vi "elevatorStuffs.vi"   [LabVIEW 2014]
uses:
  Support Files/ElevatorStates.ctl
  Support Files/DropStates.ctl
  Support Files/RC PickupStates.ctl
  Support Files/TransitionStates.ctl
  Support Files/HandOffStates.ctl
  Support Files/FeederModeStates.ctl
  Support Files/FeederModePickUpStates.ctl
  Support Files/FeederModeStartStates.ctl
  Support Files/Global Data!!!.vi
types:
  T1 = typedef "ElevatorStates.ctl" = enum16{"DropSequence", "Reset", "Drop1Stage", "2StageEngage", "Lift1Stage", "1StageEngage", "Rest", "InterruptedLift", "Manual", "Auto2Man", "Initialize", "FeederMode"}
  T2 = typedef "DropStates.ctl" = enum16{"Lower", "Retract", "Release", "Drop1Inch", "Not", "Reset", "Pause", "isArmOut", "putArmOut"}
  T3 = typedef "RC PickupStates.ctl" = enum16{"PickToteUp", "Disengage", "Drop", "Hold", "Lift", "Engage1Stage", "Rest", "DropAgain", "Done", "Lift.5", "Pause4Jones"}
  T4 = typedef "TransitionStates.ctl" = enum16{"Release 2 Stage", "Hand-Off", "Do Nothing"}
  T5 = typedef "HandOffStates.ctl" = enum16{"Done", "Release2Stage", "Engage1Stage", "Raise1Stage", "Pause"}
  T6 = typedef "FeederModePickUpStates.ctl" = enum16{"ToEnding", "Pick Up", "Engage", "DropDown", "Release", "Drop", "Wait", "Engage2Stage", "Disengage2Stage"}
  T7 = typedef "FeederModeStates.ctl" = enum16{"Ending", "PickUp", "Starting", "Reset"}
  T8 = typedef "FeederModeStartStates.ctl" = enum16{"ToPickUp", "LiftUp", "Engage", "Wait", "Lift", "Release", "Drop"}
  T9 = typedef "WPI_SwitchDevRef.ctl" = cluster{"DevStatus":errorcluster, "DIO Channel":T10, "Controller":T11, "CntIndex":T12, "Normally Closed":bool}
  T10 = typedef "FPGA_DIOChannel.ctl" = enum8{"DIO 0", "DIO 1", "DIO 2", "DIO 3", "DIO 4", "DIO 5", "DIO 6", "DIO 7", "DIO 8", "DIO 9", "DIO MXP 0", "DIO MXP 1", "DIO MXP 2", "DIO MXP 3", "DIO MXP 4", "DIO MXP 5", "DIO MXP 6", "DIO MXP 7", "DIO MXP 8", "DIO MXP 9", "DIO MXP 10", "DIO MXP 11", "DIO MXP 12", "DIO MXP 13", "DIO MXP 14", "DIO MXP 15", "Invalid"}
  T11 = typedef "FPGA_TypedefDigitalModule.ctl" = enum16{"Controller 1"}
  T12 = typedef "FPGA_CounterCtrSystemIndex.ctl" = enum8{"Ctr 0", "Ctr 1", "Ctr 2", "Ctr 3", "Ctr 4", "Ctr 5", "Ctr 6", "Ctr 7", "Invalid"}
  T13 = typedef "WPI_EncoderDevRef.ctl" = cluster{"DevStatus":errorcluster, "EncoderIndex":T14, "CounterIndex":T12, "DistancePerCount":dbl, "Decoding Type":T15}
  T14 = typedef "FPGA_EncoderIdx.ctl" = enum8{"Enc 0", "Enc 1", "Enc 2", "Enc 3", "Enc 4", "Enc 5", "Enc 6", "Enc 7", "Invalid"}
  T15 = typedef "WPI_EncoderType.ctl" = enum16{"1x", "2x", "4x"}
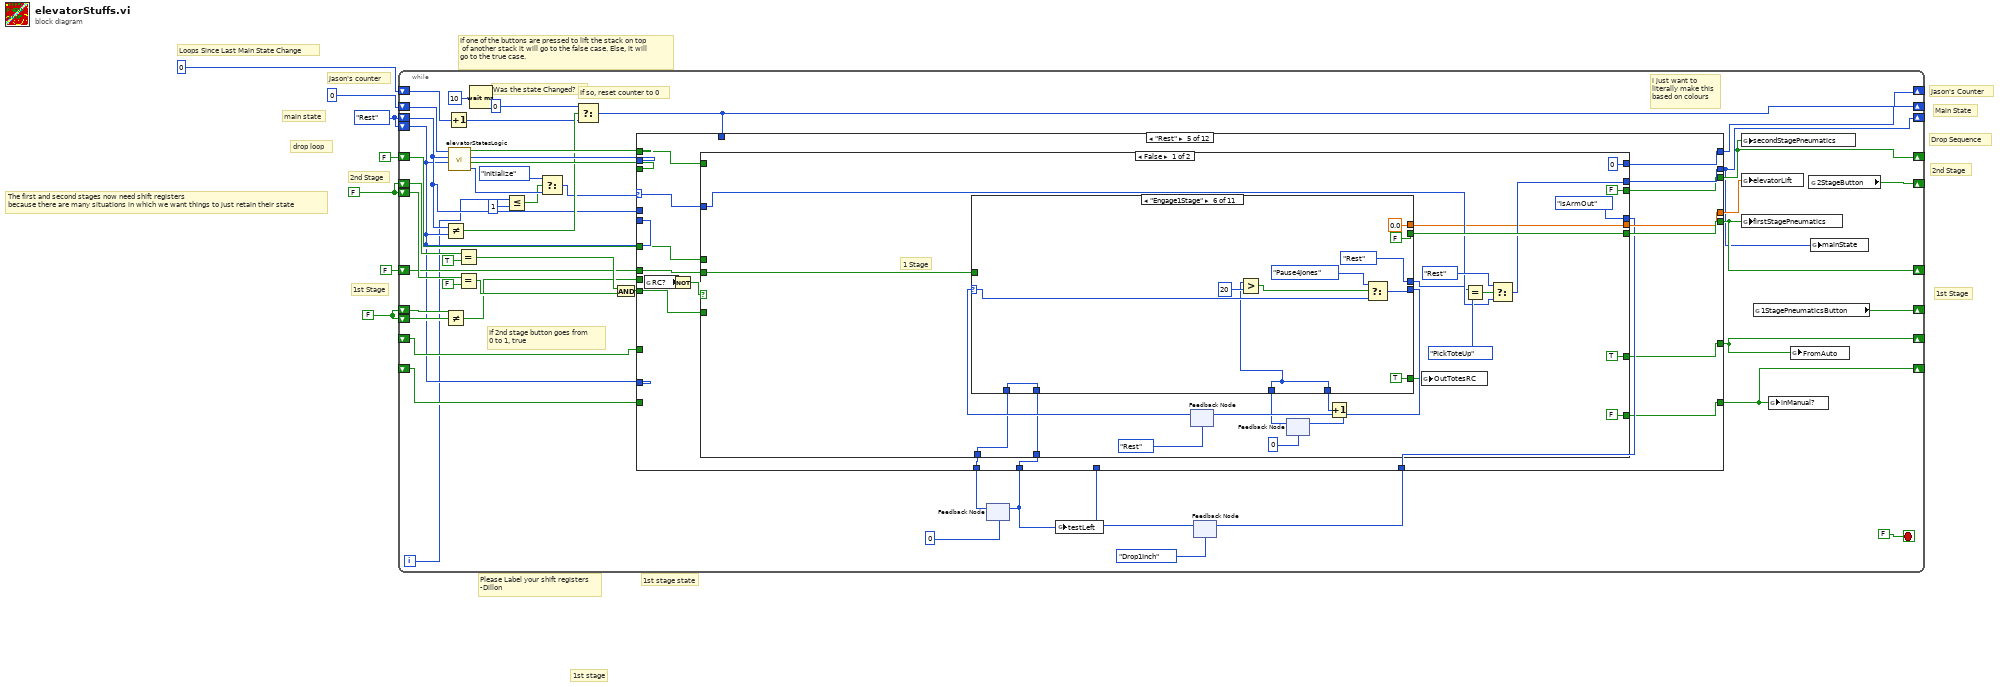
[diagram p0: block diagram]
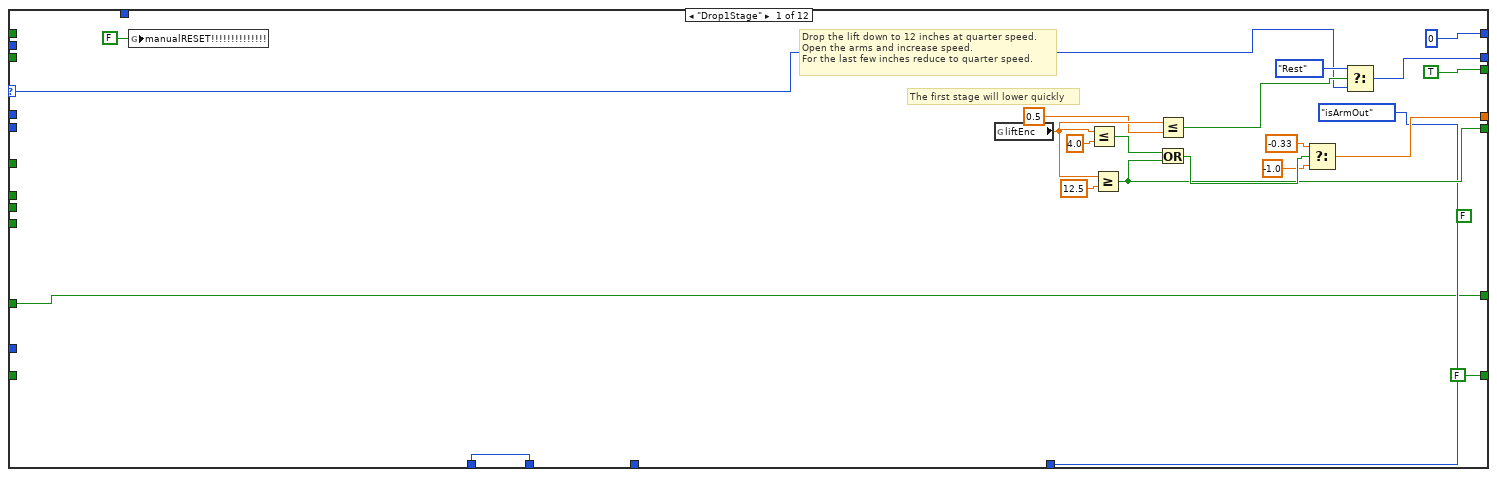
[diagram p2: hidden frame]
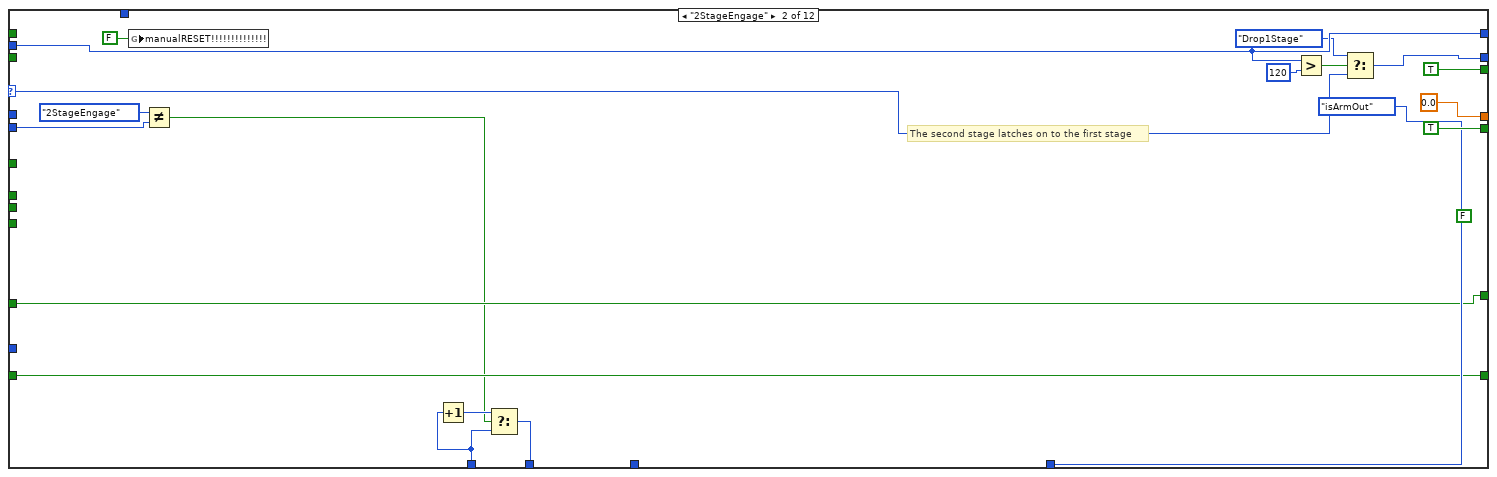
[diagram p3: hidden frame]
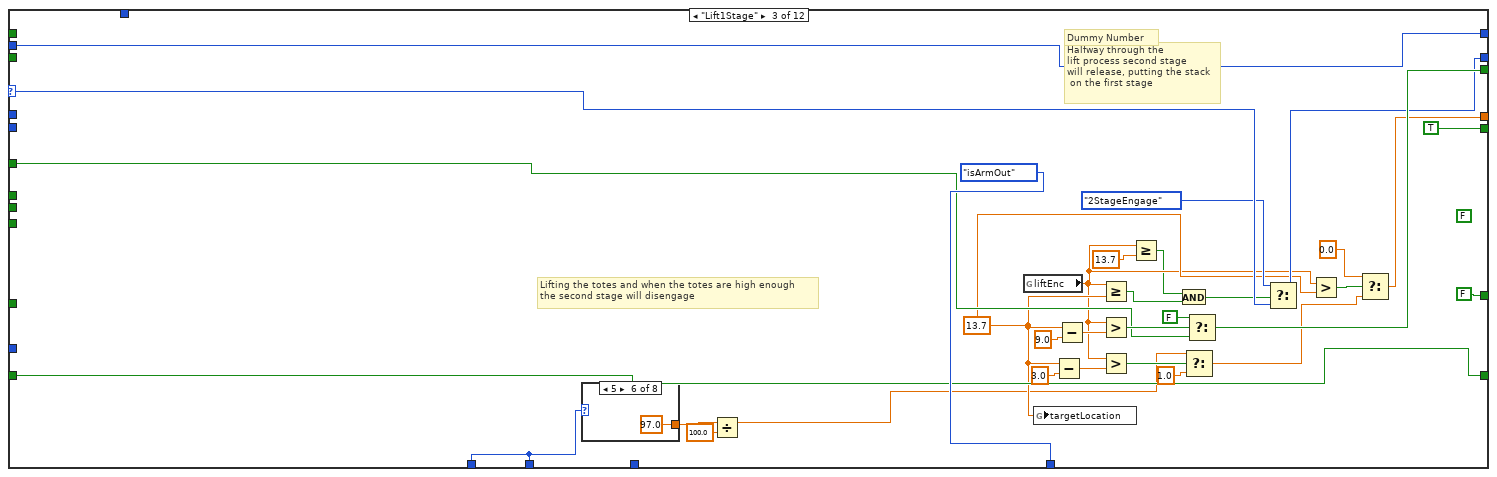
[diagram p4: hidden frame]
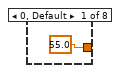
[diagram p5: hidden frame]
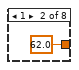
[diagram p6: hidden frame]
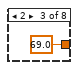
[diagram p7: hidden frame]
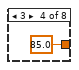
[diagram p8: hidden frame]
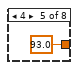
[diagram p9: hidden frame]
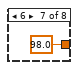
[diagram p10: hidden frame]
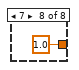
[diagram p11: hidden frame]
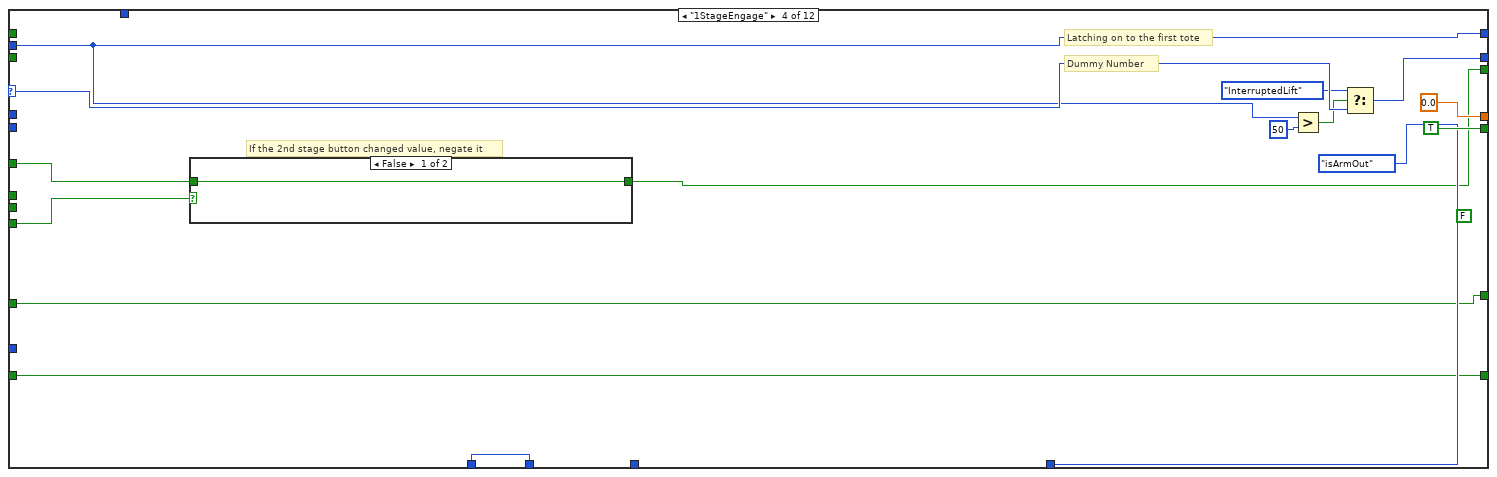
[diagram p12: hidden frame]
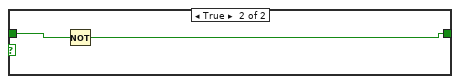
[diagram p13: hidden frame]
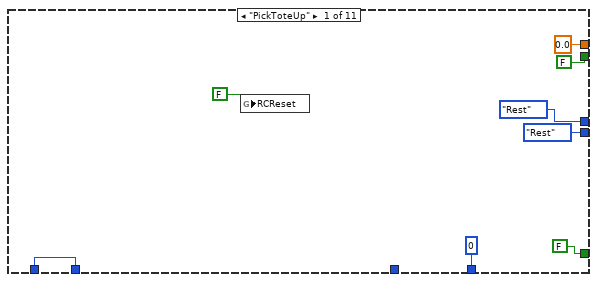
[diagram p14: hidden frame]
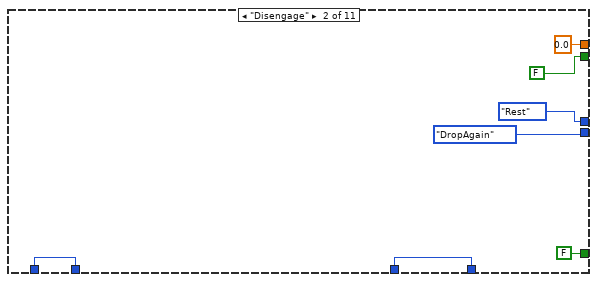
[diagram p15: hidden frame]
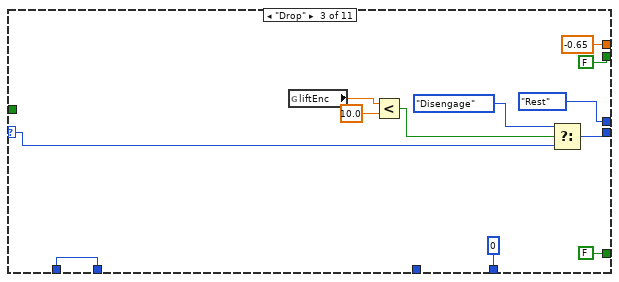
[diagram p16: hidden frame]
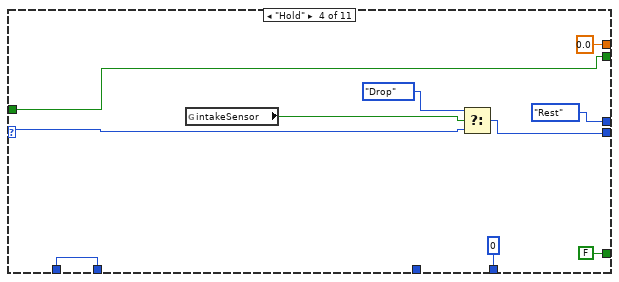
[diagram p17: hidden frame]
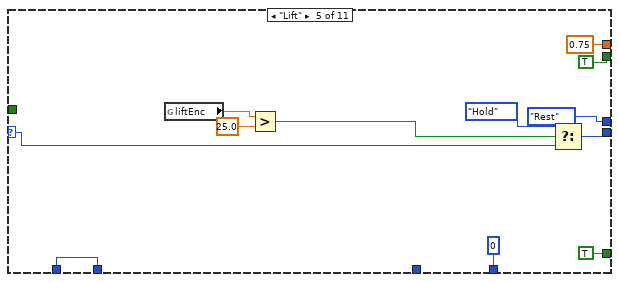
[diagram p18: hidden frame]
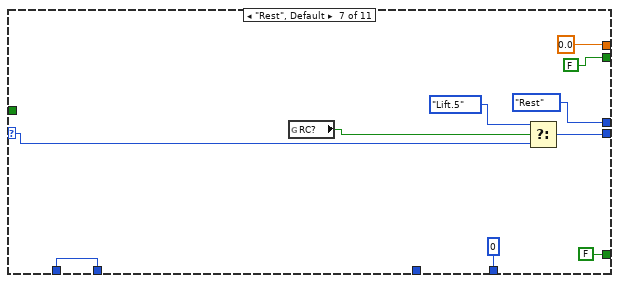
[diagram p19: hidden frame]
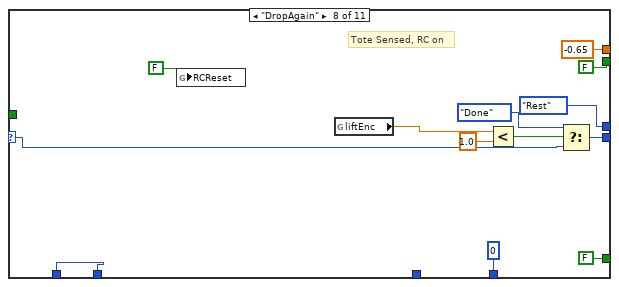
[diagram p20: hidden frame]
diagram:
  w1 = FALSE ("1StagePneumaticsButton")
  w3 = FALSE ("2StageButton")
  w6 = ElevatorStates."Rest" ("Enum")
  # "Jason's Counter"
  # "Main State"
  # "Drop Sequence"
  # "The first and second stages now need shift registers\nbecause there are many situations in which we want things to just retain their state"
  # "main state"
  # "drop loop"
  # "2nd Stage"
  # "1st Stage"
  # "1st Stage"
  # "1st stage state"
  # "1st stage"
  # "2nd Stage"
  # "Jason's counter"
  # "Loops Since Last Main State Change"
  # "Please Label your shift registers\n-Dillon"
  # "If one of the buttons are pressed to lift the stack on top\n of another stack it will go to the false case. Else, it will\ngo to the true case."
  n1 = while {
    shift-right: [w23] -> _
    shift-left: w6 -> [w15]
    shift-right: [w53] -> _
    shift-left: 0 -> [w55]
    shift-left: w6 -> [w14]
    shift-right: [w27] -> _
    shift-left: 0 -> [w44]
    shift-right: [w43] -> _
    shift-left: FALSE ("t") -> [w42]
    shift-right: [w41] -> _
    shift-left: w3 -> [w40]
    shift-left: w3 -> [w36]
    shift-right: [w33] -> _
    shift-left: FALSE ("f") -> [w28]
    shift-right: [w32] -> _
    shift-left: w1 -> [w31]
    shift-left: w1 -> [w30]
    shift-right: [w22] -> _
    shift-left: _ -> [w21]
    shift-right: [w20] -> _
    shift-left: _ -> [w19]
    i -> [w9]
    stop <- FALSE stop-if-true
    # "If 2nd stage button goes from\n0 to 1, true"
    # "If so, reset counter to 0"
    # "Was the state Changed?"
    # "i just want to \nliterally make this\nbased on colours"
    n2 = Not Equal?(x=w15, y=w14) -> (x != y?=w47:bool)
    n3 = Not Equal?(x=w31, y=w30) -> (x != y?=w29:bool)
    n4 = Increment(x=w44) -> (x+1=w45:i32)
    n5 = call "elevatorStatesLogic.vi"("oldState"=w14, "newState"=w15, "timer"=w55) -> ("State"=w12:T1, "manual?"=w48:bool, "Numeric"=w54:i32, "elevatorActive"=w49:bool)  [unwired: 5 in]
    n6 = Equal?(x=w40, y=TRUE) -> (x = y?=w38:bool)
    n7 = Equal?(x=w36, y=FALSE) -> (x = y?=w37:bool)
    n8 = Wait (ms)(milliseconds to wait=u32 10) -> ()  [unwired: 1 out]
    n9 = Less Or Equal?(x=w9, y=1) -> (x <= y?=w10:bool)
    n10 = Select(t=ElevatorStates."Initialize", s=w10, f=w12) -> (s? t:f=w13:T1)
    n11 = Select(t=0, s=w47, f=w45) -> (s? t:f=w27:i32)
    n12 = And(x=w38, y=w37) -> (x .and. y?=w39:bool)
    n13 = feedback #1(0) -> (w17:i32)
    n14 = feedback #2(DropStates."Drop1Inch" ("Enum")) -> (w25:T2)
    n15 = case shown="\"Rest\"" w13 {
      selector: w13 -> [w72 w92 w122 w148 w161 w337 w357 w399 w440 w561 _ w673]
      tunnel: [w71 w89 w120 w143 w167 w336 w367 w411 w432 w562 ElevatorStates."Rest" ("Enum") w672] -> w23
      tunnel: [w70 0.0 w108 0.0 w169 w335 w365 w386 w442 w552 0.0 ("f") w670] -> w52
      tunnel: [w62 TRUE TRUE TRUE w170 w332 TRUE ("t") w376 w439 w551 FALSE ("Stage1?") w669] -> w33
      tunnel: [TRUE TRUE ("t") w125 w139 w164 FALSE ("t") w345 FALSE ("t") FALSE ("t") w548 FALSE ("t") w652] -> w43
      tunnel: w54 -> [_ w91 w123 w145 _ _ _ _ w436 w550 _ _]
      tunnel: [0 ("t") w91 w123 w145 w168 0 ("t") 0 ("t") 0 ("t") w437 w546 0 ("Numeric") 0 ("Numeric")] -> w53
      tunnel: w49 -> [_ _ _ _ w166 _ _ _ _ _ _ _]
      tunnel: w25 -> [_ _ _ _ _ _ _ _ w441 w558 _ _]
      tunnel: [DropStates."isArmOut" ("Enum") DropStates."isArmOut" ("Enum") DropStates."isArmOut" ("Enum") DropStates."isArmOut" ("Enum") w165 DropStates."isArmOut" ("Enum") DropStates."isArmOut" ("Enum") DropStates."isArmOut" ("Enum") w438 w558 DropStates."isArmOut" ("Enum") DropStates."isArmOut" ("Enum")] -> w24
      tunnel: w48 -> [_ _ _ _ _ _ _ w385 _ _ _ _]
      tunnel: w14 -> [_ _ _ _ _ _ _ w383 _ _ _ _]
      tunnel: w42 -> [_ _ w112 w141 w163 _ w345 w379 _ _ _ _]
      tunnel: w39 -> [_ _ _ w140 w162 _ _ w380 w430 _ _ _]
      tunnel: w29 -> [_ _ _ _ _ _ _ w378 _ _ _ _]
      tunnel: w28 -> [_ _ _ _ w158 w332 _ w377 _ _ _ _]
      tunnel: w27 -> [_ _ _ _ _ _ _ _ w429 _ _ _]
      tunnel: [FALSE w84 w111 w138 w160 FALSE w348 TRUE w428 w559 FALSE FALSE] -> w22
      tunnel: w21 -> [_ w84 w111 w138 _ _ w348 _ w428 w559 _ _]
      tunnel: [w57 w83 FALSE w137 w159 FALSE TRUE w374 FALSE w539 TRUE FALSE] -> w20
      tunnel: w19 -> [w57 w83 _ w137 _ _ _ w374 _ _ _ _]
      tunnel: w17 -> [w56 w81 w99 w136 w155 w329 w346 w373 _ w547 w644 w682]
      tunnel: [w56 w79 w99 w136 w154 w329 w346 w373 0 w547 w644 w682] -> w16
      tunnel: w15 -> [_ _ _ _ _ _ _ _ _ _ _ _]
      tunnel: w14 -> [_ w77 _ _ _ _ _ _ _ _ _ _]
      frame "Drop1Stage" {
        (unwired) FALSE
        # "Drop the lift down to 12 inches at quarter speed.\nOpen the arms and increase speed.\nFor the last few inches reduce to quarter speed."
        # "The first stage will lower quickly"
        n16 = global write "Global Data!!!.vi" "manualRESET!!!!!!!!!!!!!!"(FALSE ("secondStagePneumatics")) -> ()
        n17 = global read "Global Data!!!.vi" "liftEnc"() -> (w67:dbl)
        n18 = Less Or Equal?(x=w67, y=4.0) -> (x <= y?=w65:bool)
        n19 = Greater Or Equal?(x=w67, y=12.5) -> (x >= y?=w62:bool)
        n20 = Less Or Equal?(x=w67, y=0.5) -> (x <= y?=w74:bool)
        n21 = Or(x=w65, y=w62) -> (x .or. y?=w64:bool)
        n22 = Select(t=-0.33, s=w64, f=-1.0) -> (s? t:f=w70:dbl)
        n23 = Select(t=ElevatorStates."Rest", s=w74, f=w72) -> (s? t:f=w71:T1)
      }
      frame "2StageEngage" {
        (unwired) FALSE
        # "The second stage latches on to the first stage"
        n24 = global write "Global Data!!!.vi" "manualRESET!!!!!!!!!!!!!!"(FALSE ("secondStagePneumatics")) -> ()
        n25 = Not Equal?(x=ElevatorStates."2StageEngage", y=w77) -> (x != y?=w80:bool)
        n26 = Increment(x=w81) -> (x+1=w82:i32)
        n27 = Select(t=w82, s=w80, f=w81) -> (s? t:f=w79:i32)
        n28 = Greater?(x=w91, y=120) -> (0:w88:bool)
        n29 = Select(t=ElevatorStates."Drop1Stage" ("Enum"), s=w88, f=w92) -> (s? t:f=w89:T1)
      }
      frame "Lift1Stage" {
        (unwired) FALSE
        w105 = 13.7 ("y")
        # "Halfway through the\nlift process second stage\nwill release, putting the stack\n on the first stage"
        # "Lifting the totes and when the totes are high enough\nthe second stage will disengage"
        # "Dummy Number"
        n30 = case shown="5" w99 {
          tunnel: [55.0 ("y") 62.0 ("y") 69.0 ("y") 85.0 ("y") 93.0 ("y") 97.0 ("y") 98.0 ("y") 1.0 ("y")] -> w98
          frame 0, Default {
          }
          frame 1 {
          }
          frame 2 {
          }
          frame 3 {
          }
          frame 4 {
          }
          frame 5 {
          }
          frame 6 {
          }
          frame 7 {
          }
        }
        n31 = Divide(x=w98, y=100.0) -> (x/y=w97:dbl)
        n32 = global read "Global Data!!!.vi" "liftEnc"() -> (w104:dbl)
        n33 = global write "Global Data!!!.vi" "targetLocation"(w105) -> ()
        n34 = Subtract(x=w105, y=3.0) -> (x-y=w114:dbl)
        n35 = Subtract(x=w105, y=9.0) -> (x-y=w119:dbl)
        n36 = Greater Or Equal?(x=w104, y=w105) -> (x >= y?=w100:bool)
        n37 = Greater?(x=w104, y=w119) -> (0:w127:bool)
        n38 = Greater?(x=w104, y=w114) -> (0:w116:bool)
        n39 = Greater Or Equal?(x=w104, y=13.7) -> (x >= y?=w101:bool)
        n40 = And(x=w101, y=w100) -> (x .and. y?=w102:bool)
        n41 = Select(t=w97, s=w116, f=1.0) -> (s? t:f=w109:dbl)
        n42 = Select(t=FALSE, s=w127, f=w112) -> (s? t:f=w125:bool)
        n43 = Select(t=ElevatorStates."2StageEngage", s=w102, f=w122) -> (s? t:f=w120:T1)
        n44 = Greater?(x=w104, y=w105) -> (0:w106:bool)
        n45 = Select(t=0.0, s=w106, f=w109) -> (s? t:f=w108:dbl)
      }
      frame "1StageEngage" {
        (unwired) FALSE
        # "If the 2nd stage button changed value, negate it"
        # "Latching on to the first tote"
        # "Dummy Number"
        n46 = case shown="False" w140 {
          tunnel: w141 -> [w151 w153]
          tunnel: [w151 w152] -> w139
          frame False {
          }
          frame True {
            n47 = Not(x=w153) -> (.not. x?=w152:bool)
          }
        }
        n48 = Greater?(x=w145, y=50) -> (0:w147:bool)
        n49 = Select(t=ElevatorStates."InterruptedLift" ("Enum"), s=w147, f=w148) -> (s? t:f=w143:T1)
      }
      frame "Rest" {
        n50 = global read "Global Data!!!.vi" "RC?"() -> (w157:bool)
        n51 = Not(x=w157) -> (.not. x?=w156:bool)
        n52 = case shown="False" w156 {
          tunnel: [w193 FALSE] -> w170
          tunnel: [w180 0.0] -> w169
          tunnel: [0 ("t") 0 ("t")] -> w168
          tunnel: [w183 w319] -> w167
          tunnel: w166 -> [_ w318]
          tunnel: [DropStates."isArmOut" ("Enum") DropStates."isArmOut" ("Enum")] -> w165
          tunnel: [FALSE ("t") w307] -> w164
          tunnel: w163 -> [_ w307]
          tunnel: w162 -> [_ _]
          tunnel: w161 -> [w184 w314]
          tunnel: [FALSE FALSE] -> w160
          tunnel: [TRUE TRUE] -> w159
          tunnel: w158 -> [w179 _]
          tunnel: w155 -> [w173 w308]
          tunnel: [w172 w308] -> w154
          frame False {
            # "1 Stage"
            n53 = feedback #3(RC_PickupStates."Rest") -> (w189:T3)
            n54 = feedback #4(0 ("t")) -> (w177:i32)
            n55 = case shown="\"Engage1Stage\"" w189 {
              selector: w189 -> [_ _ w220 w229 w241 w250 w261 w275 _ _ w299]
              tunnel: [FALSE FALSE FALSE ("Stage1?") w225 TRUE ("Stage1?") FALSE FALSE FALSE ("Stage1?") w283 FALSE ("Stage1?") TRUE ("Stage1?")] -> w193
              tunnel: [RC_PickupStates."Rest" RC_PickupStates."DropAgain" w221 w230 w242 w251 w262 w276 RC_PickupStates."Rest" RC_PickupStates."Engage1Stage" ("t") w300] -> w187
              tunnel: [0.0 0.0 -0.65 0.0 0.75 0.0 0.0 -0.65 0.0 0.0 0.0] -> w180
              tunnel: w179 -> [_ _ _ w225 _ _ _ _ w283 _ _]
              tunnel: w177 -> [_ w209 _ _ _ w244 _ _ w282 w289 w295]
              tunnel: [0 ("t") w209 0 ("t") 0 ("t") 0 ("t") w244 0 ("t") 0 ("t") w282 w289 w295] -> w176
              tunnel: [RC_PickupStates."Rest" RC_PickupStates."Rest" RC_PickupStates."Rest" RC_PickupStates."Rest" RC_PickupStates."Rest" RC_PickupStates."Rest" RC_PickupStates."Rest" RC_PickupStates."Rest" RC_PickupStates."PickToteUp" RC_PickupStates."Rest" RC_PickupStates."PickToteUp"] -> w174
              tunnel: w173 -> [w197 w205 w211 w223 w234 w245 w256 w266 w279 w291 w297]
              tunnel: [w197 w205 w211 w223 w234 w245 w256 w266 w279 w288 w297] -> w172
              tunnel: [FALSE FALSE FALSE FALSE TRUE TRUE FALSE FALSE FALSE TRUE TRUE] -> w171
              frame "PickToteUp" {
                n56 = global write "Global Data!!!.vi" "RCReset"(FALSE) -> ()
              }
              frame "Disengage" {
              }
              frame "Drop" {
                n57 = global read "Global Data!!!.vi" "liftEnc"() -> (w218:dbl)
                n58 = Less?(x=w218, y=10.0) -> (x < y?=w216:bool)
                n59 = Select(t=RC_PickupStates."Disengage", s=w216, f=w220) -> (s? t:f=w221:T3)
              }
              frame "Hold" {
                n60 = global read "Global Data!!!.vi" "intakeSensor"() -> (w231:bool)
                n61 = Select(t=RC_PickupStates."Drop", s=w231, f=w229) -> (s? t:f=w230:T3)
              }
              frame "Lift" {
                n62 = global read "Global Data!!!.vi" "liftEnc"() -> (w239:dbl)
                n63 = Greater?(x=w239, y=25.0) -> (0:w237:bool)
                n64 = Select(t=RC_PickupStates."Hold", s=w237, f=w241) -> (s? t:f=w242:T3)
              }
              frame "Engage1Stage" {
                n65 = Greater?(x=w244, y=20) -> (0:w247:bool)
                n66 = Select(t=RC_PickupStates."Pause4Jones", s=w247, f=w250) -> (s? t:f=w251:T3)
              }
              frame "Rest", Default {
                n67 = global read "Global Data!!!.vi" "RC?"() -> (w258:bool)
                n68 = Select(t=RC_PickupStates."Lift.5", s=w258, f=w261) -> (s? t:f=w262:T3)
              }
              frame "DropAgain" {
                # "Tote Sensed, RC on"
                n69 = global write "Global Data!!!.vi" "RCReset"(FALSE) -> ()
                n70 = global read "Global Data!!!.vi" "liftEnc"() -> (w272:dbl)
                n71 = Less?(x=w272, y=1.0) -> (x < y?=w273:bool)
                n72 = Select(t=RC_PickupStates."Done", s=w273, f=w275) -> (s? t:f=w276:T3)
              }
              frame "Done" {
                n73 = global write "Global Data!!!.vi" "RCReset"(TRUE) -> ()
              }
              frame "Lift.5" {
                n74 = Increment(x=w291) -> (x+1=w288:i32)
              }
              frame "Pause4Jones" {
                n75 = Greater?(x=w295, y=40) -> (0:w296:bool)
                n76 = Select(t=RC_PickupStates."Lift", s=w296, f=w299) -> (s? t:f=w300:T3)
              }
            }
            n77 = feedback-in #3(w187) -> ()
            n78 = Increment(x=w176) -> (x+1=w175:i32)
            n79 = feedback-in #4(w175) -> ()
            n80 = global write "Global Data!!!.vi" "OutTotesRC"(w171) -> ()
            n81 = Equal?(x=w174, y=RC_PickupStates."PickToteUp") -> (x = y?=w188:bool)
            n82 = Select(t=ElevatorStates."Rest" ("Enum"), s=w188, f=w184) -> (s? t:f=w183:T1)
          }
          frame True {
            # "If the 2nd stage button changed value, negate it"
            # "Waiting for tote to enter robot"
            n83 = global write "Global Data!!!.vi" "manualRESET!!!!!!!!!!!!!!"(FALSE ("secondStagePneumatics")) -> ()
            n84 = global write "Global Data!!!.vi" "OutTotesRC"(FALSE) -> ()
            n85 = global write "Global Data!!!.vi" "outTotes"(FALSE) -> ()
            n86 = global write "Global Data!!!.vi" "RCReset"(FALSE) -> ()
            n87 = global read "Global Data!!!.vi" "dropButton"() -> (w312:bool)
            n88 = Select(t=ElevatorStates."DropSequence" ("Enum"), s=w312, f=w314) -> (s? t:f=w315:T1)
            n89 = Select(t=ElevatorStates."1StageEngage" ("Enum"), s=w318, f=w315) -> (s? t:f=w319:T1)
          }
        }
      }
      frame "Reset" {
        (unwired) FALSE
        n90 = global write "Global Data!!!.vi" "manualRESET!!!!!!!!!!!!!!"(FALSE ("secondStagePneumatics")) -> ()
        n91 = call <vilib>:"WPI_SwitchRefNum Registry Get.vi"("refnum name"="bottomLimit") -> ("error out"=w328:errorcluster, "SwitchDevRef"=w327:T9)  [unwired: 9 in]
        n92 = call <vilib>:"WPI_SwitchGetLimitValue.vi"("error in (no error)"=w328, "SwitchDevRef"=w327) -> ("Switch Pressed"=w325:bool)  [unwired: 7 in, 2 out]
        n93 = case shown="True" w325 {
          frame False {
          }
          frame True {
            n94 = call <vilib>:"WPI_EncoderRefNum Registry Get.vi"("refnum name"="liftEnc") -> ("error out"=w344:errorcluster, "EncoderDevRef"=w343:T13)  [unwired: 9 in]
            n95 = call <vilib>:"WPI_EncoderReset.vi"("error in (no error)"=w344, "EncoderDevRef"=w343) -> ()  [unwired: 8 in, 2 out]
          }
        }
        n96 = Select(t=0.0, s=w325, f=-0.5) -> (s? t:f=w335:dbl)
        n97 = Select(t=ElevatorStates."Rest" ("Enum"), s=w325, f=w337) -> (s? t:f=w336:T1)
      }
      frame "InterruptedLift" {
        (unwired) FALSE
        w361 = 2.75 ("y")
        # "Go to new and improved\ndrop sequence"
        # "If the 2nd stage button changed value, negate it"
        n98 = global write "Global Data!!!.vi" "manualRESET!!!!!!!!!!!!!!"(FALSE ("secondStagePneumatics")) -> ()
        n99 = global read "Global Data!!!.vi" "dropButton"() -> (w356:bool)
        n100 = global read "Global Data!!!.vi" "liftEnc"() -> (w353:dbl)
        n101 = Select(t=ElevatorStates."DropSequence", s=w356, f=w357) -> (s? t:f=w359:T1)
        n102 = global write "Global Data!!!.vi" "targetLocation"(w361) -> ()
        n103 = Greater?(x=w353, y=0.5) -> (0:w351:bool)
        n104 = Greater?(x=w353, y=w361) -> (0:w355:bool)
        n105 = global read "Global Data!!!.vi" "interruptUp"() -> (w363:bool)
        n106 = Select(t=0.5, s=w351, f=1.0) -> (s? t:f=w354:dbl)
        n107 = Select(t=0.0, s=w355, f=w354) -> (s? t:f=w365:dbl)
        n108 = Select(t=ElevatorStates."Lift1Stage", s=w363, f=w359) -> (s? t:f=w367:T1)
      }
      frame "Manual" {
        (unwired) FALSE
        # "Maintain state of 2nd stage until button press"
        # "Maintain state of 1st stage until button change val"
        n109 = case shown="False" w380 {
          tunnel: w379 -> [w416 w418]
          tunnel: [w416 w417] -> _
          frame False {
          }
          frame True {
            n110 = Not(x=w418) -> (.not. x?=w417:bool)
          }
        }
        n111 = case shown="False" w378 {
          tunnel: w377 -> [w413 w415]
          tunnel: [w413 w414] -> w376
          frame False {
          }
          frame True {
            n112 = Not(x=w415) -> (.not. x?=w414:bool)
          }
        }
        n113 = Not Equal?(x=w383, y=ElevatorStates."Manual") -> (x != y?=w381:bool)
        n114 = global write "Global Data!!!.vi" "manualElevatorReLevel?"(w381) -> ()
        n115 = global read "Global Data!!!.vi" "desiredEncoderValue"() -> (w384:dbl)
        n116 = global read "Global Data!!!.vi" "liftEnc"() -> (w391:dbl)
        n117 = global write "Global Data!!!.vi" "targetLocation"(w384) -> ()
        n118 = Add(x=w384, y=0.5) -> (x+y=w396:dbl)
        n119 = Subtract(x=w391, y=w384) -> (x-y=w390:dbl)
        n120 = Greater?(x=w391, y=w396) -> (0:w409:bool)
        n121 = Subtract(x=w384, y=0.5) -> (x-y=w394:dbl)
        n122 = Less?(x=w391, y=w394) -> (x < y?=w407:bool)
        n123 = Absolute Value(x=w390) -> (abs(x)=w389:dbl)
        n124 = Select(t=0, s=w409, f=1) -> (s? t:f=w408:i32)
        n125 = Less?(x=w389, y=3.0) -> (x < y?=w387:bool)
        n126 = Select(t=2, s=w407, f=w408) -> (s? t:f=w406:i32)
        n127 = case shown="1, Default" w406 {
          tunnel: [-1.0 0.0 1.0] -> w392
          tunnel: w391 -> [_ _ _]
          tunnel: w394 -> [_ _ _]
          frame 0 {
            # "Down"
          }
          frame 1, Default {
            # "No Movement"
          }
          frame 2 {
            # "Up"
          }
        }
        n128 = global write "Global Data!!!.vi" "manualElevatorReLevel?"(FALSE ("manualElevatorReLevel?")) -> ()
        n129 = global write "Global Data!!!.vi" "resetDesired"(FALSE ("manualElevatorReLevel?")) -> ()
        n130 = global read "Global Data!!!.vi" "dropButton"() -> (w397:bool)
        n131 = Select(t=ElevatorStates."DropSequence", s=w397, f=w399) -> (s? t:f=w400:T1)
        n132 = Not(x=w385) -> (.not. x?=w405:bool)
        n133 = case shown="True" w387 {
          tunnel: w392 -> [w419 w422]
          tunnel: [w419 w420] -> w386
          frame False {
          }
          frame True {
            n134 = Multiply(x=w422, y=0.25) -> (x*y=w420:dbl)
          }
        }
        n135 = Select(t=ElevatorStates."Rest", s=w405, f=w400) -> (s? t:f=w411:T1)
      }
      frame "DropSequence" {
        (unwired) FALSE
        n136 = case shown="\"isArmOut\", Default" w441 {
          selector: w441 -> [w456 _ w474 w491 _ w506 w510 _ _]
          tunnel: [w450 0.0 0.0 -0.35 0.0 0.0 ("f") 0.0 ("f") 0.0 ("f") 0.0 ("f")] -> w442
          tunnel: w440 -> [w451 w465 w469 w488 w497 _ w511 w523 w529]
          tunnel: [w451 w465 w469 w488 w497 ElevatorStates."Reset" ("t") w511 w523 w529] -> w433
          tunnel: [FALSE ("f") FALSE ("f") FALSE TRUE ("f") FALSE FALSE ("f") FALSE ("f") TRUE ("f") TRUE ("f")] -> w439
          tunnel: [w457 DropStates."Lower" ("t") w475 w489 DropStates."Reset" ("Enum") w506 w512 DropStates."Drop1Inch" ("Enum") DropStates."Drop1Inch" ("Enum")] -> w438
          tunnel: [0 0 w471 0 0 0 w514 w522 w533] -> w437
          tunnel: w436 -> [_ _ w472 _ _ _ w514 w522 w533]
          tunnel: [FALSE FALSE FALSE FALSE FALSE TRUE FALSE FALSE FALSE] -> w434
          tunnel: w430 -> [_ _ _ _ _ _ _ _ _]
          tunnel: w429 -> [_ _ _ _ _ _ _ _ w528]
          frame "Lower" {
            n137 = global read "Global Data!!!.vi" "manual?"() -> (w443:bool)
            n138 = global write "Global Data!!!.vi" "manualElevatorReLevel?"(w443) -> ()
            n139 = global read "Global Data!!!.vi" "liftEnc"() -> (w454:dbl)
            n140 = global read "Global Data!!!.vi" "liftEnc"() -> (w448:dbl)
            n141 = Less?(x=w454, y=2.0) -> (x < y?=w452:bool)
            n142 = Less?(x=w448, y=6.0) -> (x < y?=w447:bool)
            n143 = Select(t=-0.4, s=w447, f=-1.0) -> (s? t:f=w450:dbl)
            n144 = Select(t=DropStates."Not", s=w452, f=w456) -> (s? t:f=w457:T2)
          }
          frame "Retract" {
            n145 = Wait (ms)(milliseconds to wait=u32 1000) -> ()  [unwired: 1 out]
          }
          frame "Release" {
            n146 = Increment(x=w472) -> (x+1=w471:i32)
            n147 = Greater?(x=w471, y=200) -> (0:w467:bool)
            n148 = Select(t=DropStates."Retract", s=w467, f=w474) -> (s? t:f=w475:T2)
          }
          frame "Drop1Inch" {
            w481 = 0.25 ("y")
            # "When trying to drop totes from interrupt up\nthe motor would stall trying to reach a negative\nvalue when dropping the lift."
            n149 = global read "Global Data!!!.vi" "manual?"() -> (w478:bool)
            n150 = global read "Global Data!!!.vi" "desiredEncoderValue"() -> (w483:dbl)
            n151 = global write "Global Data!!!.vi" "manualRESET!!!!!!!!!!!!!!"(w478) -> ()
            n152 = Subtract(x=w483, y=4.0) -> (x-y=w482:dbl)
            n153 = Less Or Equal?(x=w482, y=w481) -> (x <= y?=w480:bool)
            n154 = Select(t=w481, s=w480, f=w482) -> (s? t:f=w479:dbl)
            n155 = global read "Global Data!!!.vi" "liftEnc"() -> (w494:dbl)
            n156 = Less Or Equal?(x=w494, y=w479) -> (x <= y?=w493:bool)
            n157 = Select(t=DropStates."Release", s=w493, f=w491) -> (s? t:f=w489:T2)
          }
          frame "Not" {
            n158 = global write "Global Data!!!.vi" "manualRESET!!!!!!!!!!!!!!"(FALSE ("0 3")) -> ()
            n159 = global write "Global Data!!!.vi" "manualElevatorReLevel?"(FALSE ("0 3")) -> ()
            n160 = global write "Global Data!!!.vi" "outTotes"(FALSE ("outTotes")) -> ()
          }
          frame "Reset" {
          }
          frame "Pause" {
            n161 = Greater?(x=w514, y=20) -> (0:w515:bool)
            n162 = Select(t=DropStates."Lower" ("Enum"), s=w515, f=w510) -> (s? t:f=w512:T2)
          }
          frame "isArmOut", Default {
            # "1 millisecond, 2 milliseconds, 3milliseconds, ah ha ha."
            # "2nd stage should continue to do\nwhat it was doing"
            # "Otherwise we need to put the arm out"
            # "Still want the drop sequence"
            # "Assume we have\ntotes or bins"
          }
          frame "putArmOut" {
            # "Put the arm out for some amount of time."
            # "outTotes Muh Goats.\nI.E. put the arm out."
            n163 = Greater?(x=w528, y=250) -> ()  [unwired: 1 out]
          }
        }
        n164 = Select(t=ElevatorStates."Reset", s=w434, f=w433) -> (s? t:f=w432:T1)
      }
      frame "Auto2Man" {
        # "1Stage"
        # "2Stage"
        n165 = global read "Global Data!!!.vi" "Stage1?"() -> (w549:bool)
        n166 = global read "Global Data!!!.vi" "Stage2?"() -> (w538:bool)
        n167 = And(x=w549, y=w538) -> (x .and. y?=w556:bool)
        n168 = Select(t=TransitionStates."Release 2 Stage", s=w556, f=TransitionStates."Do Nothing") -> (s? t:f=w557:T4)
        n169 = Select(t=TransitionStates."Hand-Off", s=w538, f=w557) -> (s? t:f=w534:T4)
        n170 = feedback #5(TransitionStates."Do Nothing") -> (w537:T4)
        n171 = case shown="\"Hand-Off\"" w537 {
          selector: w537 -> [w563 _ _]
          tunnel: [0.0 ("f") w586 0.0 ("f")] -> w552
          tunnel: [w572 w585 w642] -> w551
          tunnel: w550 -> [w566 _ _]
          tunnel: w549 -> [w572 _ w642]
          tunnel: [FALSE w584 FALSE] -> w548
          tunnel: [w566 0 ("Numeric") 0 ("Numeric")] -> w546
          tunnel: [HandOffStates."Pause" w578 HandOffStates."Pause"] -> w545
          tunnel: [w565 FALSE w636] -> w542
          tunnel: HandOffStates."Raise1Stage" -> [_ w576 _]
          tunnel: [w563 TransitionStates."Hand-Off" w635] -> w536
          tunnel: w534 -> [_ _ w635]
          frame "Release 2 Stage", Default {
            (unwired) 0 ("Numeric")
            n172 = Greater?(x=w566, y=50) -> (0:w569:bool)
            n173 = Select(t=TRUE, s=w569, f=FALSE) -> (s? t:f=w565:bool)
          }
          frame "Hand-Off" {
            n174 = feedback #6(w576) -> (w578:T5)
            n175 = feedback #7(0 ("Numeric")) -> (w582:i32)
            n176 = case shown="\"Done\"" w578 {
              selector: w578 -> [w591 _ w608 _ w634]
              tunnel: [w593 HandOffStates."Raise1Stage" w607 HandOffStates."Pause" ("t") w633] -> w574
              tunnel: [0.0 ("f") 0.0 ("f") 0.0 ("f") 0.0 ("f") w620] -> w586
              tunnel: [TRUE TRUE TRUE TRUE FALSE] -> w585
              tunnel: [TRUE FALSE FALSE TRUE TRUE] -> w584
              tunnel: w582 -> [w592 _ w603 _ _]
              tunnel: [w592 0 ("Numeric") w603 0 ("Numeric") 0 ("Numeric")] -> w581
              frame "Pause", Default {
                n177 = Greater?(x=w592, y=100) -> (0:w594:bool)
                n178 = Select(t=HandOffStates."Release2Stage", s=w594, f=w591) -> (s? t:f=w593:T5)
              }
              frame "Done" {
              }
              frame "Release2Stage" {
                n179 = global write "Global Data!!!.vi" "manualElevatorReLevel?"(TRUE ("manualElevatorReLevel?")) -> ()
                n180 = global write "Global Data!!!.vi" "resetDesired"(TRUE ("manualElevatorReLevel?")) -> ()
                n181 = Greater?(x=w603, y=100) -> (0:w609:bool)
                n182 = Select(t=HandOffStates."Done", s=w609, f=w608) -> (s? t:f=w607:T5)
              }
              frame "Engage1Stage" {
              }
              frame "Raise1Stage" {
                n183 = global read "Global Data!!!.vi" "liftEnc"() -> (w622:dbl)
                n184 = Greater?(x=w622, y=13.0) -> (0:w631:bool)
                n185 = Greater?(x=w622, y=5.0) -> (0:w628:bool)
                n186 = Select(t=0.5, s=w628, f=1.0) -> (s? t:f=w623:dbl)
                n187 = Greater?(x=w622, y=11.0) -> (0:w624:bool)
                n188 = Select(t=0.4, s=w624, f=w623) -> (s? t:f=w620:dbl)
                n189 = Select(t=HandOffStates."Engage1Stage", s=w631, f=w634) -> (s? t:f=w633:T5)
              }
            }
            n190 = feedback-in #6(w574) -> ()
            n191 = Increment(x=w581) -> (x+1=w580:i32)
            n192 = feedback-in #7(w580) -> ()
          }
          frame "Do Nothing" {
            (unwired) 0 ("Numeric")
            n193 = Equal?(x=TransitionStates."Do Nothing", y=w635) -> (x = y?=w636:bool)
          }
        }
        n194 = feedback-in #5(w536) -> ()
        n195 = Equal?(x=w545, y=HandOffStates."Done") -> (x = y?=w543:bool)
        n196 = Compound Arithmetic op=OR(w543, w542) -> (w540:bool)
        n197 = Select(t=ElevatorStates."Manual", s=w540, f=w561) -> (s? t:f=w562:T1)
        n198 = Not(x=w540) -> (.not. x?=w539:bool)
      }
      frame "Initialize" {
        (unwired) FALSE
      }
      frame "FeederMode" {
        n199 = feedback #8(FeederModeStates."Starting") -> (w661:T7)
        n200 = feedback #9(0) -> (w667:i32)
        n201 = Increment(x=w667) -> (x+1=w665:i32)
        n202 = feedback #10(FeederModePickUpStates."Wait") -> (w659:T6)
        n203 = case shown="\"PickUp\"" w661 {
          selector: w661 -> [w711 w724 w825 w900]
          tunnel: [w711 w724 w825 w900] -> w675
          tunnel: w673 -> [_ _ _ _]
          tunnel: [w712 w728 w830 w901] -> w676
          tunnel: [-0.75 w722 w824 0.0] -> w670
          tunnel: [w700 w721 w823 FALSE] -> w669
          tunnel: w665 -> [_ _ _ w894]
          tunnel: [0 0 0 w894] -> w666
          tunnel: [w699 w717 w816 w892] -> w656
          tunnel: w659 -> [w699 w716 w816 w892]
          tunnel: [FALSE ("t") w715 FALSE ("t") FALSE ("t")] -> w652
          frame "Ending", Default {
            n204 = global read "Global Data!!!.vi" "liftEnc"() -> (w710:dbl)
            n205 = Less?(x=w710, y=0.3) -> (x < y?=w708:bool)
            n206 = global read "Global Data!!!.vi" "liftEnc"() -> (w704:dbl)
            n207 = Less?(x=w704, y=25.0) -> (x < y?=w703:bool)
            n208 = Select(t=FALSE, s=w703, f=TRUE) -> (s? t:f=w700:bool)
            n209 = Select(t=4.0, s=w708, f=3.0) -> (s? t:f=w712:dbl)
          }
          frame "PickUp" {
            (unwired) 0
            n210 = feedback #11(0) -> (w718:i32)
            n211 = Increment(x=w718) -> (x+1=w726:i32)
            n212 = case shown="\"Wait\"" w716 {
              selector: w716 -> [_ w743 w754 w763 w770 w781 w796 w800 w810]
              tunnel: w726 -> [_ _ w751 _ w769 _ w788 w804 w808]
              tunnel: [0 0 w751 0 w769 0 w788 w804 w808] -> w725
              tunnel: [FeederModePickUpStates."Drop" w744 w755 w760 w772 w779 w791 w802 w811] -> w717
              tunnel: [0.0 1.0 0.0 -0.5 0.0 -0.5 0.0 0.0 0.0] -> w722
              tunnel: [TRUE TRUE TRUE FALSE FALSE TRUE TRUE TRUE TRUE] -> w721
              tunnel: [FALSE ("t") FALSE ("t") FALSE ("t") FALSE ("t") FALSE ("t") FALSE ("t") FALSE ("t") TRUE ("t") FALSE ("t")] -> w715
              frame "ToEnding", Default {
              }
              frame "Pick Up" {
                (unwired) 0
                n213 = global write "Global Data!!!.vi" "FeederMode?"(FALSE ("FeederMode?")) -> ()
                n214 = global read "Global Data!!!.vi" "liftEnc"() -> (w746:dbl)
                n215 = Greater?(x=w746, y=28.5) -> (0:w740:bool)
                n216 = Select(t=FeederModePickUpStates."Wait", s=w740, f=w743) -> (s? t:f=w744:T6)
              }
              frame "Engage" {
                n217 = Greater?(x=w751, y=50) -> (0:w750:bool)
                n218 = Select(t=FeederModePickUpStates."Pick Up", s=w750, f=w754) -> (s? t:f=w755:T6)
              }
              frame "DropDown" {
                n219 = global read "Global Data!!!.vi" "liftEnc"() -> (w765:dbl)
                n220 = Less?(x=w765, y=11.7) -> (x < y?=w762:bool)
                n221 = Select(t=FeederModePickUpStates."Engage", s=w762, f=w763) -> (s? t:f=w760:T6)
              }
              frame "Release" {
                # "Just change the first stage"
                n222 = Greater?(x=w769, y=50) -> (0:w767:bool)
                n223 = Select(t=FeederModePickUpStates."DropDown" ("y"), s=w767, f=w770) -> (s? t:f=w772:T6)
              }
              frame "Drop" {
                n224 = global write "Global Data!!!.vi" "just to be sure"(FALSE ("just to be sure")) -> ()
                n225 = global read "Global Data!!!.vi" "liftEnc"() -> (w784:dbl)
                n226 = Less?(x=w784, y=22.0) -> (x < y?=w782:bool)
                n227 = Select(t=FeederModePickUpStates."Release", s=w782, f=w781) -> (s? t:f=w779:T6)
              }
              frame "Wait" {
                n228 = global read "Global Data!!!.vi" "interruptUp"() -> (w787:bool)
                n229 = global read "Global Data!!!.vi" "FeederMode?"() -> (w792:bool)
                n230 = Select(t=FeederModePickUpStates."Engage2Stage", s=w787, f=w796) -> (s? t:f=w794:T6)
                n231 = Select(t=FeederModePickUpStates."ToEnding", s=w792, f=w794) -> (s? t:f=w791:T6)
              }
              frame "Engage2Stage" {
                n232 = Greater?(x=w804, y=50) -> (0:w801:bool)
                n233 = Select(t=FeederModePickUpStates."Disengage2Stage", s=w801, f=w800) -> (s? t:f=w802:T6)
              }
              frame "Disengage2Stage" {
                n234 = Greater?(x=w808, y=65) -> (0:w806:bool)
                n235 = Select(t=FeederModePickUpStates."Drop", s=w806, f=w810) -> (s? t:f=w811:T6)
              }
            }
            n236 = feedback-in #11(w725) -> ()
            n237 = Equal?(x=w717, y=FeederModePickUpStates."ToEnding") -> (x = y?=w719:bool)
            n238 = Select(t=3.0, s=w719, f=2.0) -> (s? t:f=w728:dbl)
          }
          frame "Starting" {
            n239 = feedback #12(0) -> (w828:i32)
            n240 = feedback #13(FeederModeStartStates."Drop") -> (w834:T8)
            n241 = case shown="\"ToPickUp\", Default" w834 {
              selector: w834 -> [_ w847 w857 w864 w869 w877 w889]
              tunnel: [FeederModeStartStates."ToPickUp" w848 w856 w861 w870 w881 w890] -> w819
              tunnel: w828 -> [_ _ w853 _ _ w879 _]
              tunnel: [0 0 w853 0 0 w879 0] -> w827
              tunnel: [0.0 1.0 0.2 0.0 1.0 0.0 -0.5] -> w824
              tunnel: [TRUE TRUE TRUE FALSE FALSE FALSE TRUE] -> w823
              frame "ToPickUp", Default {
                n242 = global write "Global Data!!!.vi" "just to be sure"(FALSE ("just to be sure")) -> ()
              }
              frame "LiftUp" {
                n243 = global read "Global Data!!!.vi" "liftEnc"() -> (w845:dbl)
                n244 = Greater?(x=w845, y=30.0) -> (0:w843:bool)
                n245 = Select(t=FeederModeStartStates."ToPickUp", s=w843, f=w847) -> (s? t:f=w848:T8)
              }
              frame "Engage" {
                n246 = Greater?(x=w853, y=50) -> (0:w854:bool)
                n247 = Select(t=FeederModeStartStates."LiftUp", s=w854, f=w857) -> (s? t:f=w856:T8)
              }
              frame "Wait" {
                # "This is just Button A"
                n248 = global read "Global Data!!!.vi" "interruptUp"() -> (w862:bool)
                n249 = Select(t=FeederModeStartStates."Engage", s=w862, f=w864) -> (s? t:f=w861:T8)
              }
              frame "Lift" {
                n250 = global read "Global Data!!!.vi" "liftEnc"() -> (w872:dbl)
                n251 = Greater?(x=w872, y=8.0) -> (0:w867:bool)
                n252 = Select(t=FeederModeStartStates."Wait", s=w867, f=w869) -> (s? t:f=w870:T8)
              }
              frame "Release" {
                n253 = Greater?(x=w879, y=50) -> (0:w880:bool)
                n254 = Select(t=FeederModeStartStates."Lift", s=w880, f=w877) -> (s? t:f=w881:T8)
              }
              frame "Drop" {
                n255 = global read "Global Data!!!.vi" "liftEnc"() -> (w887:dbl)
                n256 = Less?(x=w887, y=0.3) -> (x < y?=w885:bool)
                n257 = Select(t=FeederModeStartStates."Release", s=w885, f=w889) -> (s? t:f=w890:T8)
              }
            }
            n258 = Increment(x=w827) -> (x+1=w826:i32)
            n259 = feedback-in #12(w826) -> ()
            n260 = global write "Global Data!!!.vi" "ResetFeederMode"(FALSE ("ResetFeederMode")) -> ()
            n261 = Equal?(x=w819, y=FeederModeStartStates."ToPickUp") -> (x = y?=w820:bool)
            n262 = Select(t=2.0, s=w820, f=1.0) -> (s? t:f=w830:dbl)
            n263 = Select(t=FeederModeStartStates."Drop", s=w820, f=w819) -> (s? t:f=w817:T8)
            n264 = feedback-in #13(w817) -> ()
          }
          frame "Reset" {
            n265 = Greater?(x=w894, y=3) -> (0:w895:bool)
            n266 = Select(t=5.0, s=w895, f=4.0) -> (s? t:f=w901:dbl)
          }
        }
        n267 = feedback-in #9(w666) -> ()
        n268 = case shown="5" w676 {
          tunnel: w675 -> [_ _ _ _ _]
          tunnel: [FeederModeStates."Starting" FeederModeStates."PickUp" FeederModeStates."Ending" FeederModeStates."Reset" FeederModeStates."Starting"] -> w664
          tunnel: [FALSE FALSE FALSE FALSE TRUE] -> w671
          tunnel: [FALSE ("ResetFeederMode") FALSE ("ResetFeederMode") FALSE ("ResetFeederMode") FALSE ("ResetFeederMode") TRUE ("ResetFeederMode")] -> w662
          frame 1, Default {
          }
          frame 2 {
          }
          frame 3 {
          }
          frame 4 {
          }
          frame 5 {
          }
        }
        n269 = Select(t=FeederModeStates."Starting", s=w662, f=w664) -> (s? t:f=w655:T7)
        n270 = feedback-in #8(w655) -> ()
        n271 = Equal?(x=FeederModeStates."Starting" ("t"), y=w655) -> (x = y?=w657:bool)
        n272 = Select(t=FeederModePickUpStates."Wait", s=w657, f=w656) -> (s? t:f=w653:T6)
        n273 = feedback-in #10(w653) -> ()
        n274 = Select(t=ElevatorStates."Rest", s=w671, f=w673) -> (s? t:f=w672:T1)
      }
    }
    n275 = feedback-in #1(w16) -> ()
    n276 = global write "Global Data!!!.vi" "testLeft"(w16) -> ()
    n277 = feedback-in #2(w24) -> ()
    n278 = global write "Global Data!!!.vi" "secondStagePneumatics"(w43) -> ()
    n279 = global write "Global Data!!!.vi" "elevatorLift"(w52) -> ()
    n280 = global write "Global Data!!!.vi" "firstStagePneumatics"(w33) -> ()
    n281 = global read "Global Data!!!.vi" "1StagePneumaticsButton"() -> (w32:bool)
    n282 = global write "Global Data!!!.vi" "inManual?"(w22) -> ()
    n283 = global write "Global Data!!!.vi" "FromAuto"(w20) -> ()
    n284 = global read "Global Data!!!.vi" "2StageButton"() -> (w41:bool)
    n285 = global write "Global Data!!!.vi" "mainState"(w23) -> ()
  }
